vi "add volume by URL.vi"(5 "volume parent dir":path, 7 "issue parent dir":path, 8 "error in (no error)":errorcluster, 10 "URL":string, 11 "ComicVine_manager in":refnum<class "ComicVine_manager.lvclass">) -> (0 "error out":errorcluster, 3 "ComicVine_manager out":refnum<class "ComicVine_manager.lvclass">)   [LabVIEW 2024, in "ComicVine_manager.lvclass"]
uses:
  ComicVine_manager.lvclass
  ComicVine_manager.lvclass/ComicVine_manager.ctl
  comic_class/comic_class.lvclass
  series_class/series_class.lvclass
  C:/Code/LabVIEW_Projects/applications/ComicVine_API/comic_class/comic_class.lvclass
  C:/Code/LabVIEW_Projects/applications/ComicVine_API/series_class/series_class.lvclass
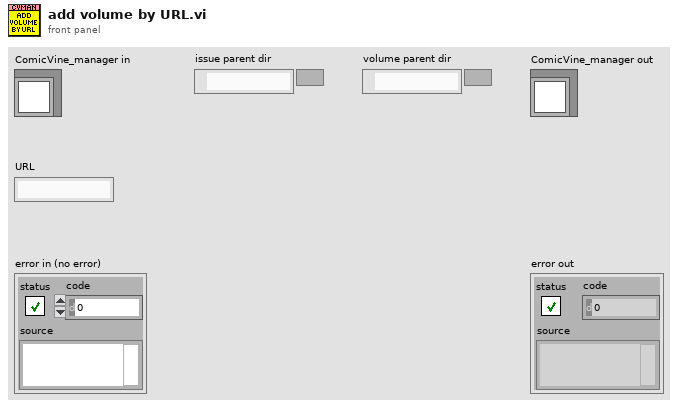
[diagram p1: front panel]
types:
  T1 = typedef "issueInfo.ctl" = cluster{"cover date":timestamp, "release date":timestamp, "number":string, "url":string, "small cover url":string, "name":string, "large cover url":string, "id":string, "creators":T2[], "characters":T3[], "teams":T4[], "locations":T5[], "concepts":T6[], "objects":T7[], "storyArcs":T8[], "description":string}
  T2 = typedef "creator.ctl" = cluster{"name":string, "role":string, "url":string}
  T3 = typedef "character.ctl" = cluster{"name":string, "url":string}
  T4 = typedef "team.ctl" = cluster{"name":string, "url":string}
  T5 = typedef "location.ctl" = cluster{"name":string, "url":string}
  T6 = typedef "concept.ctl" = cluster{"name":string, "url":string}
  T7 = typedef "thing.ctl" = cluster{"name":string, "url":string}
  T8 = typedef "storyArc.ctl" = cluster{"name":string, "url":string}
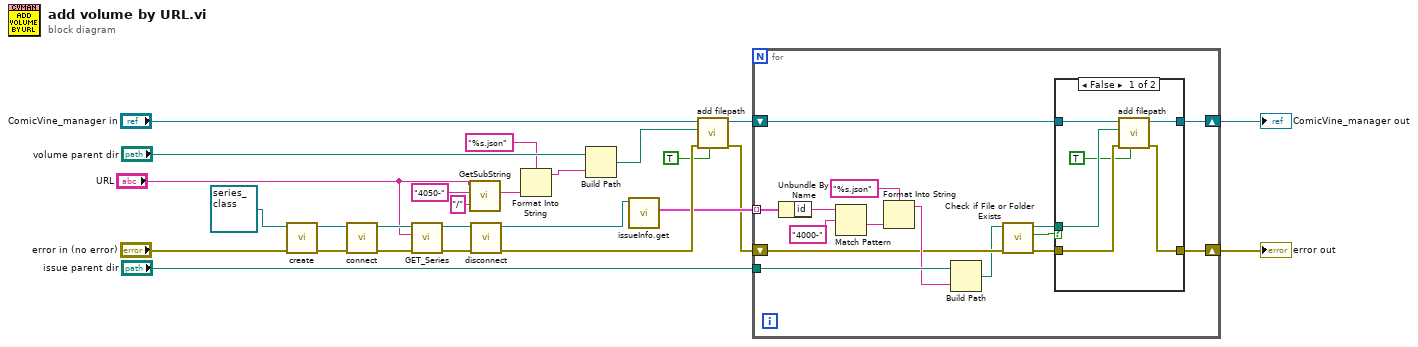
[diagram p0: block diagram]
diagram:
  n1 = call "create.vi"("error in (no error)"="error in (no error)", "comic_class in"=refnum<class "series_class.lvclass"> refnum ("series_class.lvclass")) -> ("error out"=w23:errorcluster, "comic_class out"=w24:refnum<class "series_class.lvclass">)  [unwired: 8 in]
  n2 = call-dynamic "connect.vi"("error in (no error)"=w23, "comic_class in"=w24) -> ("error out"=w21:errorcluster, "comic_class out"=w22:refnum<class "series_class.lvclass">)  [unwired: 8 in]
  n3 = call "GET_Series.vi"("error in (no error)"=w21, "series URL"="URL", "ComicVine_class in"=w22) -> ("error out"=w18:errorcluster, "ComicVine_class out"=w19:refnum<class "series_class.lvclass">)  [unwired: 7 in]
  n4 = call "GetSubString.vi"("End Search"="/", "Start Search"="4050-" ("regular expression"), "String In"="URL") -> ("Match"=w3:string)  [unwired: 6 in, 2 out]
  n5 = call-dynamic "disconnect.vi"("error in (no error)"=w18, "comic_class in"=w19) -> ("error out"=w14:errorcluster, "comic_class out"=w17:refnum<class "series_class.lvclass">)  [unwired: 8 in]
  n6 = Format Into String(format string="%s.json", w3) -> (resulting string=w1:string)  [unwired: 2 in, 1 out]
  n7 = Build Path(base path="volume parent dir", name or relative path=w1) -> (appended path=w15:path)
  n8 = call "issueInfo.get.vi"("ComicVine_class in"=w17) -> ("issueInfo"=w12:T1[])  [unwired: 9 in, 1 out]
  n9 = call "add filepath.vi"("priority (F)"=TRUE, "error in (no error)"=w14, "filepath"=w15, "ComicVine_manager in"="ComicVine_manager in") -> ("error out"=w10:errorcluster, "ComicVine_manager out"=w9:refnum<class "ComicVine_manager.lvclass">)  [unwired: 6 in]
  n10 = for {
    tunnel: w12 -> [w41] mode=indexing
    tunnel: "issue parent dir" -> [w36]
    shift-right: [w30] -> w7
    shift-left: w10 -> [w34]
    shift-right: [w28] -> w8
    shift-left: w9 -> [w29]
    n11 = Unbundle By Name(w41) -> ("id"=w40:string)
    n12 = Match Pattern(string=w40, regular expression="4000-") -> (after substring=w38:string)  [unwired: 1 in, 3 out]
    n13 = Format Into String(format string="%s.json", w38) -> (resulting string=w35:string)  [unwired: 2 in, 1 out]
    n14 = Build Path(base path=w36, name or relative path=w35) -> (appended path=w33:path)
    n15 = call <vilib>:"Check if File or Folder Exists.vi"("error in (no error)"=w34, "path"=w33) -> ("error out"=w31:errorcluster, "file or folder exists?"=w32:bool, "dup path"=w27:path)  [unwired: 7 in]
    n16 = case shown="False" w32 {
      tunnel: w31 -> [w45 w49]
      tunnel: [w44 w49] -> w30
      tunnel: [w43 w48] -> w28
      tunnel: w29 -> [w47 w48]
      tunnel: w27 -> [w46 _]
      frame False {
        n17 = call "add filepath.vi"("priority (F)"=TRUE, "error in (no error)"=w45, "filepath"=w46, "ComicVine_manager in"=w47) -> ("error out"=w44:errorcluster, "ComicVine_manager out"=w43:refnum<class "ComicVine_manager.lvclass">)  [unwired: 6 in]
      }
      frame True {
      }
    }
  }
  "error out" <- w7
  "ComicVine_manager out" <- w8
